vi "HowManyColums.vi"(8 "error in (no error)":errorcluster) -> (0 "error out":errorcluster, 3 "数目":i32)   [LabVIEW 2014]
panel:
  out "数目":string
  out "Data 2":string[][](array[string])
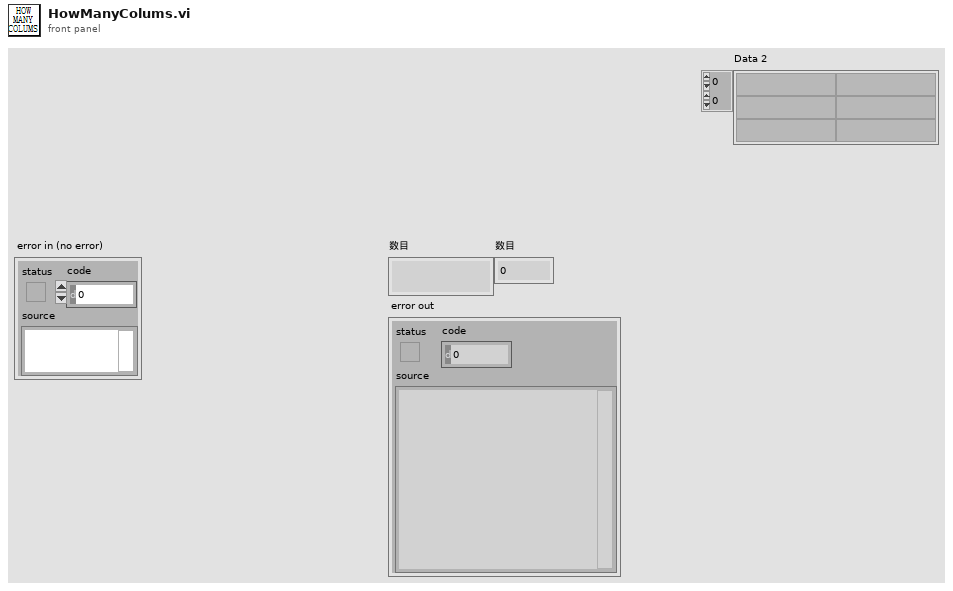
[diagram p1: front panel]
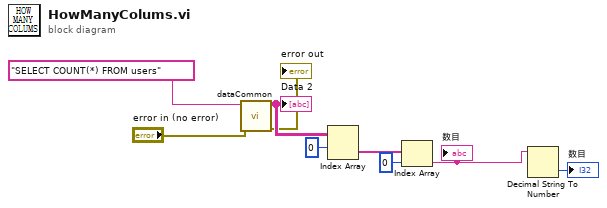
[diagram p0: block diagram]
diagram:
  n1 = call "dataCommon.vi"("error in (no error)"="error in (no error)", "Command Text"="SELECT COUNT(*) FROM users") -> ("error out"=→"error out":errorcluster, "Data"=w8:string[][])  [unwired: 8 in]
  "Data 2" <- w8
  n2 = Index Array(array=w8, index (row)=0 ("索引 (行)")) -> (element=w6:string[])  [unwired: 1 in]
  n3 = Index Array(array=w6, index=0 ("索引")) -> (element=w2:string)
  "数目" <- w2
  n4 = Decimal String To Number(string=w2) -> (number=→"数目":i32)  [unwired: 2 in, 1 out]
